vi "get runtime class name.vi"(8 "error in":errorcluster, 11 "Watchdog configuration in":refnum<class "Watchdog configuration.lvclass">) -> (0 "error out":errorcluster, 2 "class name":string, 3 "Watchdog configuration out":refnum<class "Watchdog configuration.lvclass">)   [LabVIEW 2013, in "Watchdog configuration.lvclass"]
doc: "Provides an interface for determining the module runtime class associated with this module configuration. This class name can then be used to dynamically load or locate the runtime class for initialization purposes."
uses:
  Watchdog configuration.lvclass
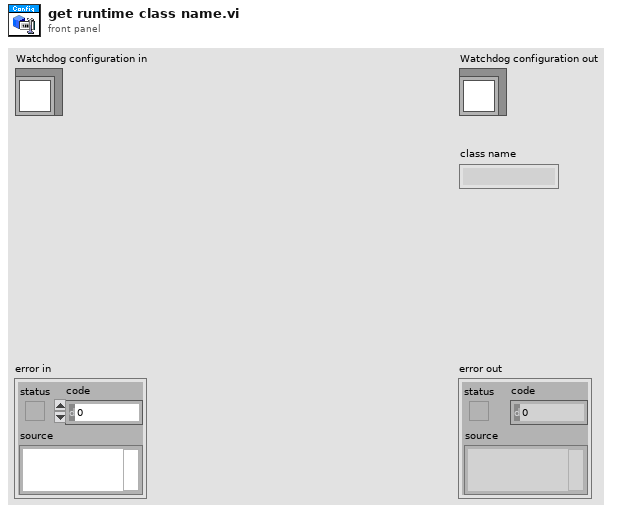
[diagram p1: front panel]
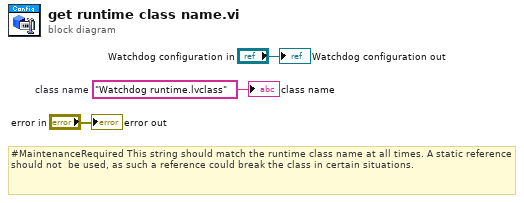
[diagram p0: block diagram]
diagram:
  w1 = "Watchdog runtime.lvclass"  # class name
  # "#MaintenanceRequired This string should match the runtime class name at all times. A static reference should not  be used, as such a reference could break the class in certain situations."
  "error out" <- "error in"
  "Watchdog configuration out" <- "Watchdog configuration in"
  "class name" <- w1
